vi "Query Scan Status.vi"(8 "error in (no error)":errorcluster, 11 "VISA resource name":refnum<visa-resource-name>) -> (0 "error out":errorcluster, 1 "Autoscan On":bool, 2 "Channel":u16(ring)=1 items=["1"=1, "2"=2, "3"=3, "4"=4, "5"=5, "6"=6, "7"=7, "8"=8, "9"=9, "10"=10, "11"=11, "12"=12, "13"=13, "14"=14, "15"=15, "16"=16], 3 "VISA resource name out":refnum<visa-resource-name>)   [LabVIEW 2015, in "Lake Shore 372.lvlib"]
doc: "Queries which channel is being scanned and if the Autoscan feature is active. Functions only when the Model 3726 Scanner is installed.\n\nNote:\nIf no scanner is installed, <B>SCAN?</B> will return a value of 1 for the active measurement input and the autoscan value will be 0, indicating OFF."
uses:
  <instrlib>/Lake Shore 372/Lake Shore 372.lvlib
  <vilib>/regexp/Match Regular Expression.xnode
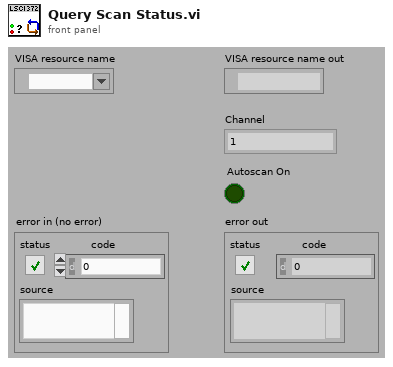
[diagram p1: front panel]
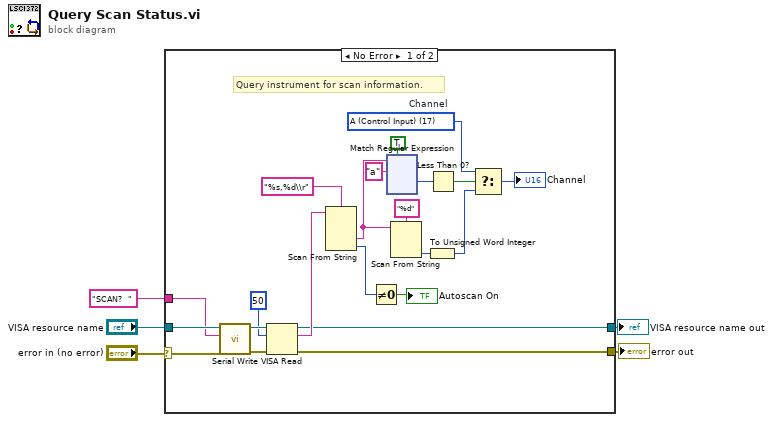
[diagram p0: block diagram]
diagram:
  n1 = case shown="No Error" "error in (no error)" {
    selector: "error in (no error)" -> [w7 w142]
    tunnel: "VISA resource name" -> [w24 w143]
    tunnel: "SCAN?  " -> [w19 _]
    tunnel: [w9 w143] -> w3
    tunnel: [w8 w142] -> w2
    frame No Error {
      w10 = u16 17 items=["1"=1, "2"=2, "3"=3, "4"=4, "5"=5, "6"=6, "7"=7, "8"=8, "9"=9, "10"=10, "11"=11, "12"=12, "13"=13, "14"=14, "15"=15, "16"=16, "A (Control Input)"=17]  # Channel
      # "Query instrument for scan information."
      n2 = call <instrlib>:"Serial Write.vi"("error in (no error)"=w7, "Write Buffer (\"\")"=w19, "VISA resource name"=w24) -> ("error out"=w26:errorcluster, "VISA resource name out"=w27:refnum<visa-resource-name>)  [unwired: 6 in, 1 out]
      n3 = VISA Read(VISA resource name=w27, byte count=50, error in (no error)=w26) -> (VISA resource name out=w9:refnum<visa-resource-name>, read buffer=w20:string, error out=w8:errorcluster)  [unwired: 1 out]
      n4 = Scan From String(format string="%s,%d\\r", input string=w20) -> (output 1=w13:string, output 2=w21:i32)  [unwired: 4 in, 3 out]
      n5 = Not Equal To 0?(x=w21) -> (x != 0?=→"Autoscan On":bool)
      n6 = xnode "Match Regular Expression"("input string"=w13, "regular expression"="a", "ignore case? (F)"=TRUE) -> ("offset past match"=w16:i32)  [unwired: 3 in, 4 out]
      n7 = Scan From String(format string="%d", input string=w13) -> (output 1=w12:i32)  [unwired: 3 in, 3 out]
      n8 = To Unsigned Word Integer(number=w12) -> (unsigned 16bit integer=w6:u16)
      n9 = Less Than 0?(x=w16) -> (x < 0?=w15:bool)
      n10 = Select(t=w10, s=w15, f=w6) -> (s? t:f=→"Channel":u16)
    }
    frame Error {
    }
  }
  "error out" <- w2
  "VISA resource name out" <- w3
